vi "test Loopback.vi"(8 "error in":errorcluster, 11 "TestCase in":refnum<class "Single Core Simple Loopback.lvclass">) -> (0 "error out":errorcluster, 3 "TestCase out":refnum<class "Single Core Simple Loopback.lvclass">)   [LabVIEW 2020, in "Single Core Simple Loopback.lvclass"]
uses:
  Single Core Simple Loopback.lvclass
  C:/Users/nitest/Desktop/Git 2020/niveristand-custom-device-testing-tools/VeriStandTestCase/VeriStandTestCase.lvclass
  <vilib>/numeric/Random Number (Range) I64.vi
  <vilib>/numeric/sub_Random U32.vi
  <vilib>/addons/_JKI Toolkits/VI Tester/TestCase.llb/TestCase.lvclass
  C:/Program Files (x86)/National Instruments/LabVIEW 2020/vi.lib/addons/_JKI Toolkits/VI Tester/TestCase.llb/TestCase.lvclass
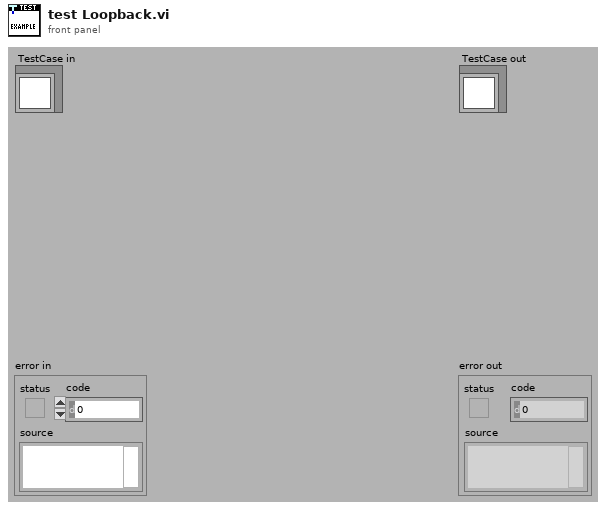
[diagram p1: front panel]
types:
  T1 = typedef "NI_VS Workspace ExecutionAPI.lvlib/WorkspaceAPI.ctl" = refnum<k24>
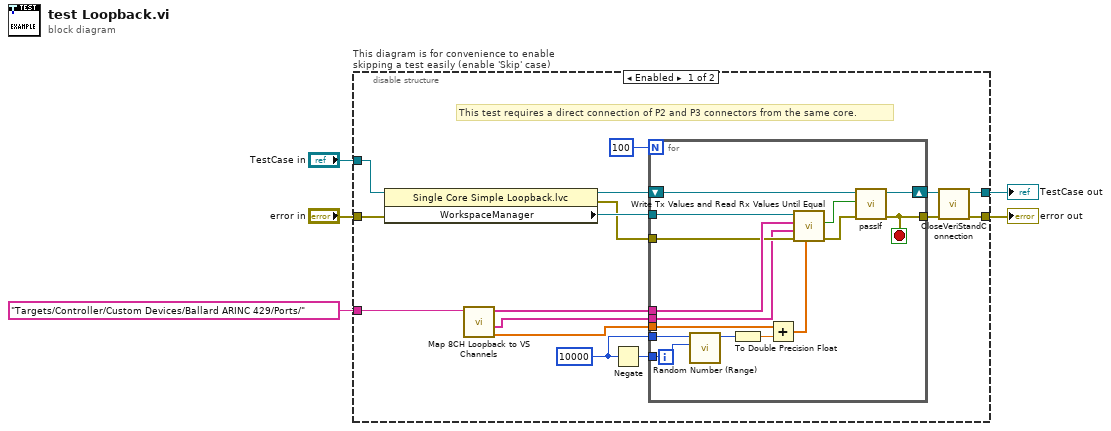
[diagram p0: block diagram]
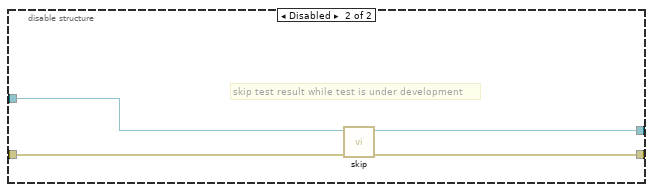
[diagram p2: hidden frame]
diagram:
  n1 = disable-structure "This diagram is for convenience to enable skipping a test easily (enable 'Skip' case)" shown="Enabled" {
    disable-tunnel: "TestCase in" -> [w7 w40]
    disable-tunnel: [w21 w38] -> w2
    disable-tunnel: [w20 w39] -> w4
    disable-tunnel: "error in" -> [w6 w37]
    disable-tunnel: "Targets/Controller/Custom Devices/Ballard ARINC 429/Ports/" ("Channel") -> [w10 _]
    frame Enabled {
      w19 = i64 10000 ("upper bound (100)")
      # "This test requires a direct connection of P2 and P3 connectors from the same core."
      n2 = property class="Single Core Simple Loopback.lvc"(reference=w7, error in=w6) -> (reference out=w14:refnum<class "Single Core Simple Loopback.lvclass">, error out=w15:errorcluster, "WorkspaceManager"=w16:T1)
      n3 = call "Map 8CH Loopback to VS Channels.vi"("Base Path to Ports"=w10) -> ("Channel Count"=w8:dbl[], "Rx Channel Array"=w9:string[], "Tx Channel Array"=w17:string[])  [unwired: 7 in, 1 out]
      n4 = Negate(x=w19) -> (-x=w18:i64)
      n5 = for {
        N: 100 -> [_]
        tunnel: w8 -> [w34]
        tunnel: w19 -> [w33]
        tunnel: w18 -> [w32]
        tunnel: w17 -> [w31]
        tunnel: w16 -> [w30]
        tunnel: w15 -> [w29]
        tunnel: w9 -> [w28]
        shift-right: [w25] -> w13
        shift-left: w14 -> [w26]
        tunnel: [w23] -> w12
        stop <- w23 stop-if-true
        n6 = call-poly <vilib>:"Random Number (Range).vi"("lower bound (-100)"=w32, "upper bound (100)"=w33) -> ("number"=w36:i64)  [unwired: 9 in]
        n7 = To Double Precision Float(number=w36) -> (double precision float=w35:dbl)
        n8 = Add(x=w34, y=w35) -> (x+y=w24:dbl[])
        n9 = call "Write Tx Values and Read Rx Values Until Equal.vi"("Tx values"=w24, "error in"=w29, "Rx aliases"=w28, "Tx aliases"=w31, "workspace manager in"=w30) -> ("error out"=w27:errorcluster, "values equal"=w22:bool)  [unwired: 4 in, 1 out]
        n10 = call-dynamic "passIf.vi"("error in (no error)"=w27, "pass"=w22, "TestCase in"=w26) -> ("error out"=w23:errorcluster, "TestCase out"=w25:refnum<class "Single Core Simple Loopback.lvclass">)  [unwired: 7 in]
      }
      n11 = call-dynamic "CloseVeriStandConnection.vi"("error in (no error)"=w12, "VeriStand Test Case in"=w13) -> ("error out"=w20:errorcluster, "VeriStand Test Case out"=w21:refnum<class "Single Core Simple Loopback.lvclass">)  [unwired: 8 in]
    }
    frame Disabled {
      # "skip test result while test is under development"
      n12 = call <vilib>:"skip.vi"("error in (no error)"=w37, "TestCase in"=w40) -> ("error out"=w39:errorcluster, "TestCase out"=w38:refnum<class "Single Core Simple Loopback.lvclass">)  [unwired: 8 in]
    }
  }
  "error out" <- w4
  "TestCase out" <- w2
